vi "Test Process Require Error Handler to be Initialized.vi"(8 "error in (no error)":errorcluster, 11 "Process Test In":refnum<class "Process Test.lvclass">) -> (0 "error out":errorcluster, 3 "Process Test Out":refnum<class "Process Test.lvclass">)   [LabVIEW 2020, in "Process Test.lvclass"]
uses:
  Process Test.lvclass
  C:/Program Files (x86)/National Instruments/LabVIEW 2020/vi.lib/Asteme/LUnit/Test Case.lvclass
  Mock Error Handler/Mock Error Handler.lvclass
  C:/Users/anton/Documents/GitHub/Triarc-Framework/source/Framework/Error Handler Interface/Error Handler Interface.lvclass
  Framework/Process/Process.lvclass/Process.ctl
  <vilib>/Asteme/LUnit/Test Case.lvclass/Test Case.ctl
  <vilib>/Asteme/LUnit/LUnit Assertion Result.lvclass/LUnit Assertion Result.ctl
  Framework/Process/Public/Get Lifecycle State.vi
  Framework/Process/Protected/Messaging/Enqueue Message.vi
  <vilib>/Utility/error.llb/Clear Errors.vi
  <vilib>/Asteme/LUnit/Palette/Fail.vi
  <vilib>/Asteme/LUnit/Palette/Pass.vi
  <vilib>/Asteme/LUnit/Set Assertion Type.vi
  <vilib>/Asteme/LUnit/Variant to string.vi
  <vilib>/AdvancedString/1D String Array to Delimited String.vi
  <vilib>/Asteme/LUnit/Add test result.vi
  <vilib>/Asteme/LUnit/LUnit Write Passed.vi
  <vilib>/Asteme/LUnit/LUnit Get Test Case.vi
  <vilib>/Asteme/LUnit/LUnit Write Message.vi
  <vilib>/Asteme/LUnit/LUnit Write Description.vi
  <vilib>/Asteme/LUnit/LUnit Write Assertion Type.vi
  <vilib>/Asteme/LUnit/Read Test Case Name.vi
  <vilib>/Utility/error.llb/Error Cluster From Error Code.vi
  <vilib>/Asteme/LUnit/Assertion Result/LUnit Get Test Name.vi
  <vilib>/Utility/Data Type/Get Type Information.vi
  <vilib>/Utility/LVClass/Get LV Class Name.vi
  Framework/Process/Process.lvclass
  <vilib>/Asteme/LUnit/LUnit Assertion Result.lvclass
  <vilib>/Asteme/LUnit/Test Case.lvclass
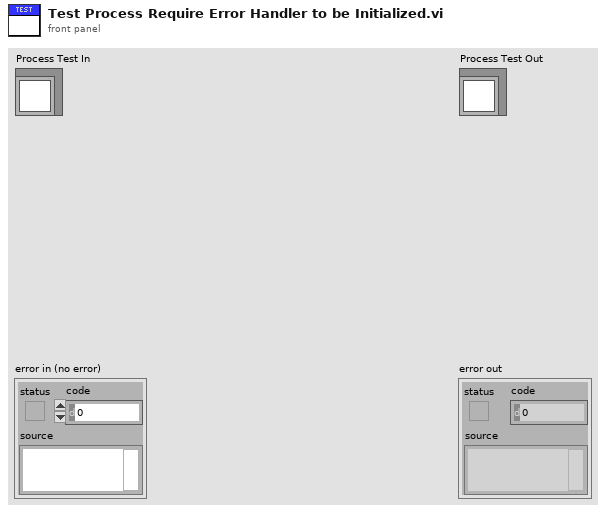
[diagram p1: front panel]
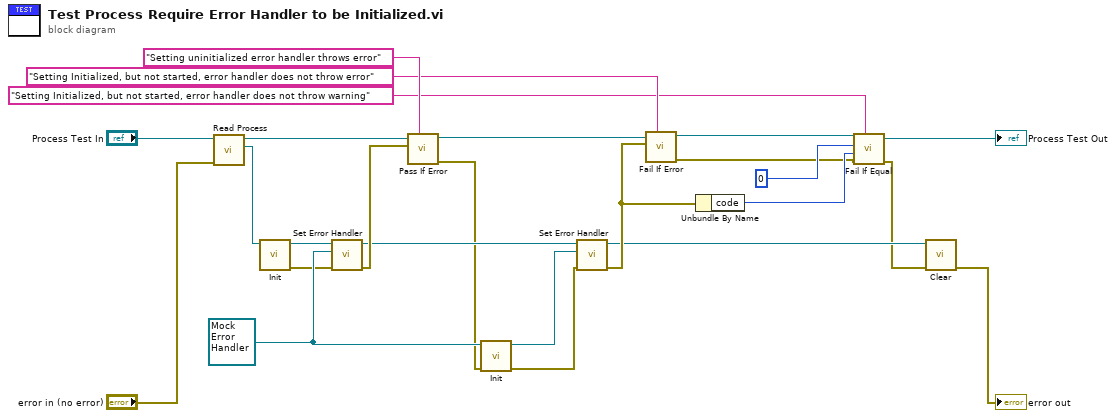
[diagram p0: block diagram]
diagram:
  w23 = refnum<class "Mock Error Handler.lvclass"> refnum ("Mock Error Handler.lvclass")
  n1 = call "Read Process.vi"("error in (no error)"="error in (no error)", "Process Test in"="Process Test In") -> ("Process.lvclass"=w24:refnum<class "Process.lvclass">, "Process Test out"=w20:refnum<class "Process Test.lvclass">)  [unwired: 7 in, 1 out]
  n2 = call-dynamic "Init.vi"("Process In"=w24) -> ("error out"=w4:errorcluster, "Process Out"=w5:refnum<class "Process.lvclass">)  [unwired: 9 in]
  n3 = call "Set Error Handler.vi"("error in (no error)"=w4, "Error Handler"=w23, "Process In"=w5) -> ("error out"=w19:errorcluster, "Process Out"=w18:refnum<class "Process.lvclass">)  [unwired: 7 in]
  n4 = call <vilib>:"Pass If Error.vi"("Description"="Setting uninitialized error handler throws error", "Assert error"=w19, "Test Case In"=w20) -> ("error out"=w17:errorcluster, "Test Case Out"=w7:refnum<class "Process Test.lvclass">)  [unwired: 7 in]
  n5 = call-dynamic "Init.vi"("error in (no error)"=w17, "Mock Error Handler In"=w23) -> ("error out"=w16:errorcluster, "Mock Error Handler Out"=w22:refnum<class "Mock Error Handler.lvclass">)  [unwired: 8 in]
  n6 = call "Set Error Handler.vi"("error in (no error)"=w16, "Error Handler"=w22, "Process In"=w18) -> ("error out"=w14:errorcluster, "Process Out"=w3:refnum<class "Process.lvclass">)  [unwired: 7 in]
  n7 = call <vilib>:"Fail If Error.vi"("Description"="Setting Initialized, but not started, error handler does not throw error", "Assert error"=w14, "Test Case In"=w7) -> ("error out"=w12:errorcluster, "Test Case Out"=w6:refnum<class "Process Test.lvclass">)  [unwired: 7 in]
  n8 = Unbundle By Name(w14) -> ("code"=w15:i32)
  n9 = call <vilib>:"Fail If Equal.vi"("Description"="Setting Initialized, but not started, error handler does not throw warning", "error in (no error)"=w12, "Actual"=w15, "Expected"=0, "Test Case In"=w6) -> ("error out"=w2:errorcluster, "Test Case Out"=→"Process Test Out":refnum<class "Process Test.lvclass">)  [unwired: 5 in]
  n10 = call-dynamic "Clear.vi"("error in (no error)"=w2, "Process In"=w3) -> ("error out"=→"error out":errorcluster)  [unwired: 8 in, 1 out]
